vi "Simple Read FTDI.vi"(8 "error In":errorcluster, 10 "Bytes To Read":u32, 11 "FTDI Handle In":u32) -> (0 "error out":errorcluster, 1 "Bytes Read":u32, 2 "Read Data":u8[](array[numeric]))   [LabVIEW 2011, in "NMR.lvclass"]
uses:
  NMR.lvclass
panel:
  out "FT_Status":u32(ring) items=["FT_OK", "FT_INVALID_HANDLE", "FT_DEVICE_NOT_FOUND", "FT_DEVICE_NOT_OPENED", "FT_IO_ERROR", "FT_INSUFFICIENT_RESOURCES", "FT_INVALID_PARAMETER", "FT_INVALID_BAUD_RATE", "FT_DEVICE_NOT_OPENED_FOR_ERASE", "FT_DEVICE_NOT_OPENED_FOR_WRITE", "FT_FAILED_TO_WRITE_DEVICE", "FT_EEPROM_READ_FAILED", "FT_EEPROM_WRITE_FAILED", "FT_EEPROM_ERASE_FAILED", "FT_EEPROM_NOT_PRESENT", "FT_EEPROM_NOT_PROGRAMMED", "FT_INVALID_ARGS", "FT_NOT_SUPPORTED", "FT_OTHER_ERROR"]
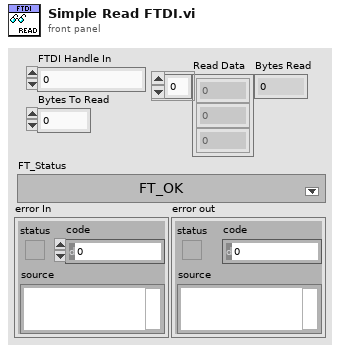
[diagram p1: front panel]
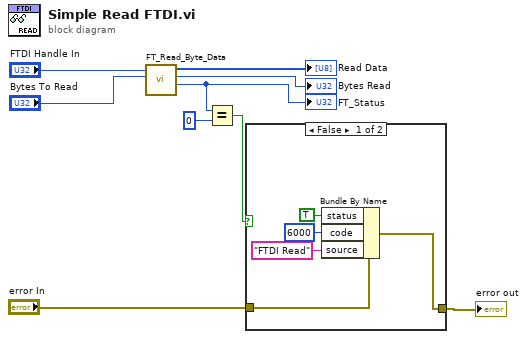
[diagram p0: block diagram]
diagram:
  n1 = call <instrlib>:"FT_Read_Byte_Data.vi"("Bytes To Read"="Bytes To Read", "Handle"="FTDI Handle In") -> ("FT_Status"=w3:u32, "Bytes Read"=→"Bytes Read":u32, "Read Data"=→"Read Data":u8[])  [unwired: 6 in, 1 out]
  "FT_Status" <- w3
  n2 = Equal?(x=w3, y=u32 0) -> (x = y?=w1:bool)
  n3 = case shown="False" w1 {
    tunnel: [w13 w15] -> w4
    tunnel: "error In" -> [w14 w15]
    frame False {
      n4 = Bundle By Name(cluster=w14, "status"=TRUE, "code"=6000, "source"="FTDI Read") -> (w13:errorcluster)
    }
    frame True {
    }
  }
  "error out" <- w4
